vi "Render EscapedVariable.vi"(8 "Error In":errorcluster) -> (0 "Error Out":errorcluster)   [LabVIEW 2018, in "Tests.lvlib" / "Render.lvlib"]
uses:
  Render.lvlib
  src/Toolkit/Readers/String/String.lvclass
  D:/Users/cfield/Code/Field R&D Services/Mustache/trunk/src/Toolkit/Readers/Abstract/Abstract.lvclass
  src/Toolkit/Render/Support/Render to String.vi
  <vilib>/addons/_JKI Toolkits/Caraya/classes/Test/Test.lvclass
  <vilib>/addons/_JKI Toolkits/Caraya/classes/Assert/Assert.lvclass
  src/Toolkit/Render/Render.lvclass
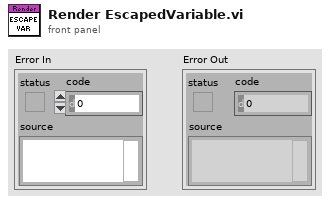
[diagram p1: front panel]
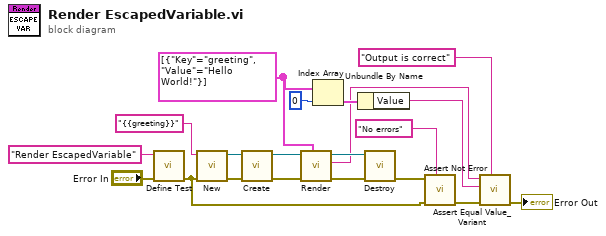
[diagram p0: block diagram]
diagram:
  w1 = cluster{"Key":string, "Value":string}[] [{"Key"="greeting", "Value"="Hello World!"}] ("Data")
  n1 = call <vilib>:"Define Test.vi"("error in (no error)"="Error In", "Label (VI Title)"="Render EscapedVariable") -> ("error out"=w18:errorcluster)  [unwired: 9 in]
  n2 = call "New.vi"("Error In"=w18, "String"="{{greeting}}" ("format string")) -> ("Error Out"=w11:errorcluster, "String"=w12:refnum<class "String.lvclass">)  [unwired: 8 in]
  n3 = call "Create.vi"("Error In"=w11, "Reader"=w12) -> ("Error Out"=w9:errorcluster, "Render"=w10:refnum<class "Render.lvclass">)  [unwired: 8 in]
  n4 = call-poly "Render.vi"("Data"=w1, "Error In"=w9, "Render In"=w10) -> ("Error Out"=w8:errorcluster, "Output"=w2:string, "Render Out"=w7:refnum<class "Render.lvclass">)  [unwired: 6 in]
  n5 = Index Array(array=w1, index=0) -> (element=w4:cluster{"Key":string, "Value":string})
  n6 = Unbundle By Name(w4) -> ("Value"=w3:string)
  n7 = call "Destroy.vi"("Error In"=w8, "Render"=w7) -> ("Error Out"=w6:errorcluster)  [unwired: 8 in, 1 out]
  n8 = call <vilib>:"Assert Not Error.vi"("Label"="No errors", "error in (no error)"=w18, "Not Error?"=w6) -> ("error out"=w16:errorcluster)  [unwired: 8 in]
  n9 = call <vilib>:"Assert Equal Value_Variant.vi"("Label"="Output is correct", "error in (no error)"=w16, "Y"=w3, "X"=w2) -> ("error out"=→"Error Out":errorcluster)  [unwired: 7 in]
